vi "Quick Laser Power Log.vi"(8 "error in (no error)":errorcluster, 11 "Digital in":refnum<vi>) -> (3 "Numeric":dbl)   [LabVIEW 2023]
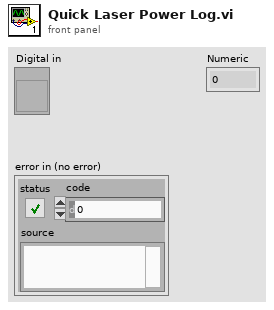
[diagram p1: front panel]
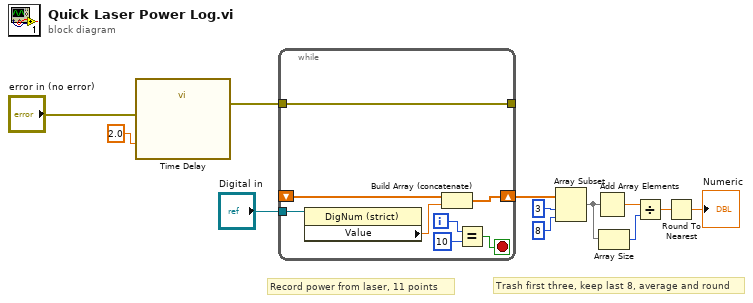
[diagram p0: block diagram]
diagram:
  # "Trash first three, keep last 8, average and round"
  # "Record power from laser, 11 points"
  n1 = call "Time Delay"("error in (no error)"="error in (no error)", "Delay Time (s)"=2.0) -> ("error out"=w10:errorcluster)  [unwired: 9 in]
  n2 = while {
    shift-right: [w20] -> w4
    shift-left: _ -> [w19]
    tunnel: [w14] -> _
    tunnel: w10 -> [w14]
    tunnel: "Digital in" -> [w13]
    i -> [w18]
    stop <- w16 stop-if-true
    n3 = property class="DigNum (strict)"(reference=w13) -> ("Value"=w15:dbl)  [unwired: 1 in, 2 out]
    n4 = Build Array (concatenate)(w19, w15) -> (w20:dbl[])
    n5 = Equal?(x=w18, y=10) -> (x = y?=w16:bool)
  }
  n6 = Array Subset(array=w4, index=3, length=8) -> (w1:dbl[])
  n7 = Add Array Elements(numeric array=w1) -> (sum=w6:dbl)
  n8 = Array Size(array=w1) -> (size(s)=w7:i32)
  n9 = Divide(x=w6, y=w7) -> (x/y=w8:dbl)
  n10 = Round To Nearest(number=w8) -> (nearest integer value=→"Numeric":dbl)
